vi "Datasheet Get Spara Result.vi"(5 "Frequency unit":string, 7 "Frequency":string, 8 "Run Information":T1, 9 "Type":T6, 10 "Format":T7=enum."SWR", 11 "Sxx":string) -> (3 "Table item":string)   [LabVIEW 2011]
uses:
  www/tests/S Parameter/TypeDefs/SP Format.ctl
  Datasheet Table Sxx Type.ctl
  TDMS/TDMS Run.ctl
  TDMS/TDMS Channel (Sxx).ctl
  database/Fields/Field Record.ctl
  database/Fields/Field DataTypes.ctl
  database/Fields/Field NextItem.ctl
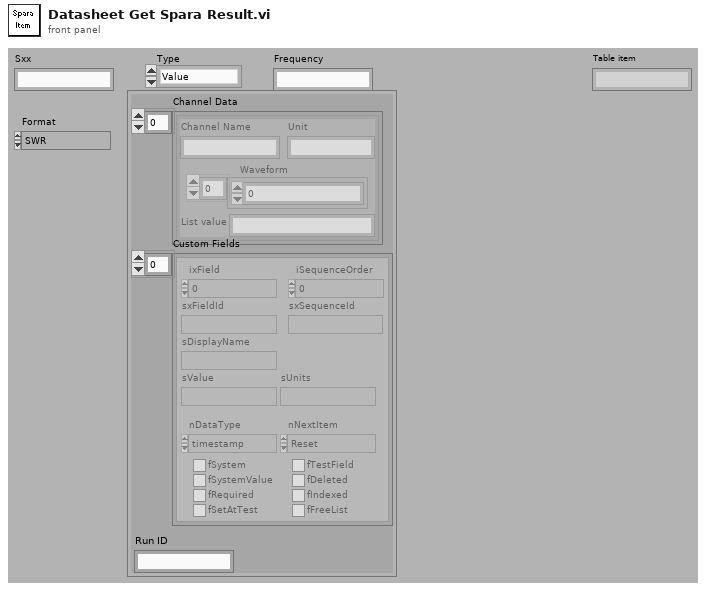
[diagram p1: front panel]
types:
  T1 = typedef "TDMS Run.ctl" = cluster{"Channel Data":T2[], "Custom Fields":T3[], "Run ID":string}
  T2 = typedef "TDMS Channel (Sxx).ctl" = cluster{"Channel Name":string, "Waveform":dbl[], "Unit":string, "List value":string}
  T3 = typedef "Field Record.ctl" = cluster{"ixField":i32, "iSequenceOrder":i32, "sxFieldId":string, "sxSequenceId":string, "sDisplayName":string, "sValue":string, "sUnits":string, "nDataType":T4, "nNextItem":T5, "fSystem":bool, "fSystemValue":bool, "fRequired":bool, "fSetAtTest":bool, "fTestField":bool, "fDeleted":bool, "fIndexed":bool, "fFreeList":bool}
  T4 = typedef "Field DataTypes.ctl" = enum32{"text", "numeric", "list", "timestamp", "boolean"}
  T5 = typedef "Field NextItem.ctl" = enum32{"Reset", "Retain", "Auto-Increment"}
  T6 = typedef "datasheet table Sxx type.ctl" = enum16{"Value", "Maximum", "Minimum", "Max Freq", "maxlimit", "minlimit", "Min Freq", "maxfreqlimit", "minfreqlimit"}
  T7 = typedef "SP Format.ctl" = enum16{"Log Mag", "Lin Mag", "SWR", "Phase", "Expanded Phase", "Delay", "Insertion Loss", "Isolation", "Return Loss"}
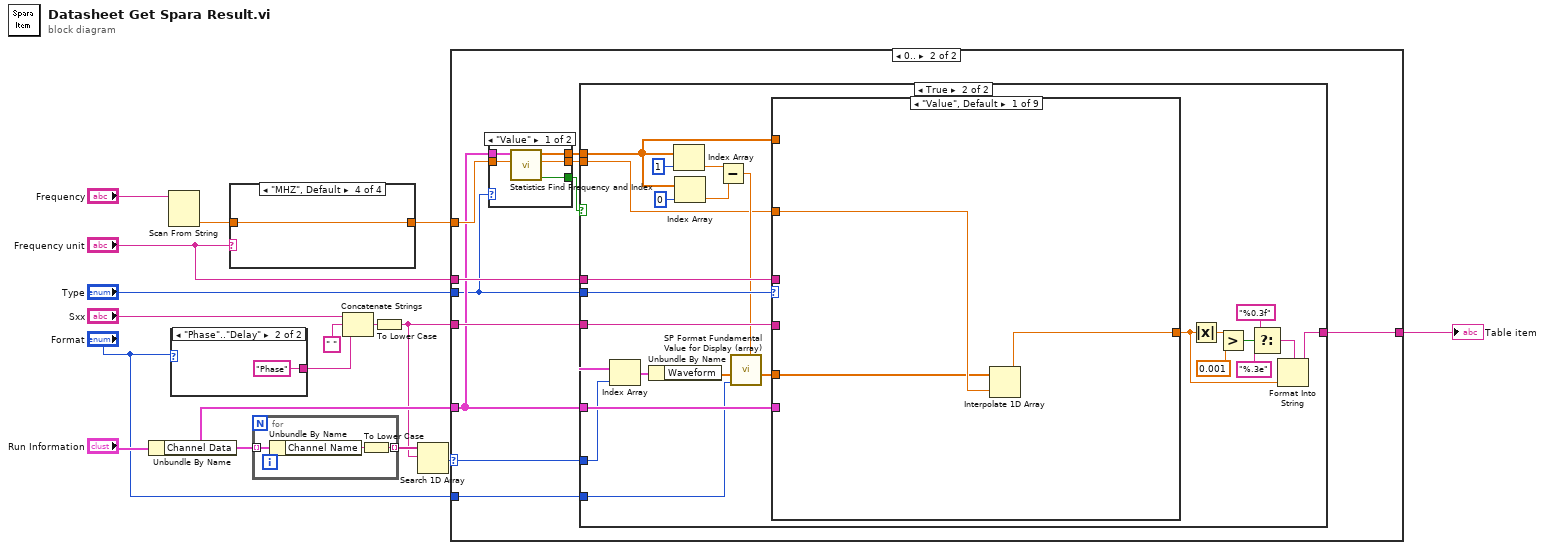
[diagram p0: block diagram]
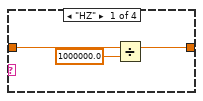
[diagram p2: hidden frame]
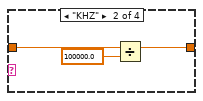
[diagram p3: hidden frame]
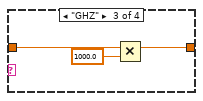
[diagram p4: hidden frame]
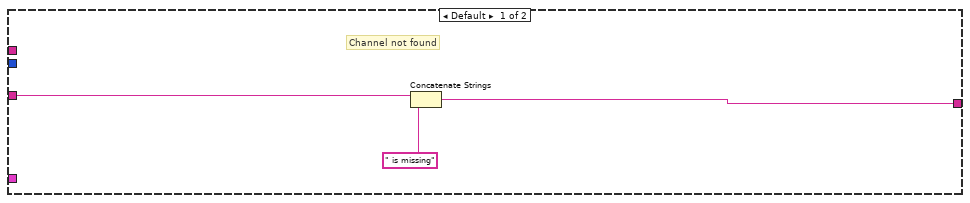
[diagram p5: hidden frame]
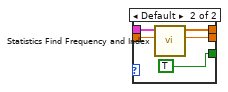
[diagram p6: hidden frame]
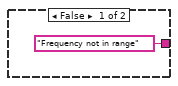
[diagram p7: hidden frame]
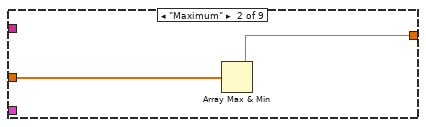
[diagram p8: hidden frame]
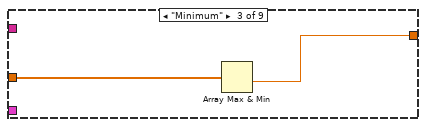
[diagram p9: hidden frame]
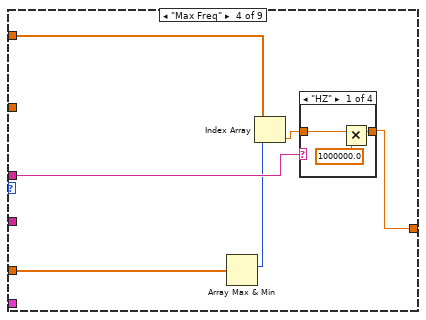
[diagram p10: hidden frame]
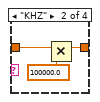
[diagram p11: hidden frame]
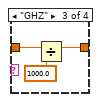
[diagram p12: hidden frame]
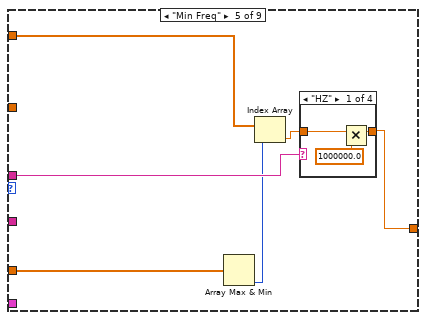
[diagram p14: hidden frame]
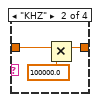
[diagram p15: hidden frame]
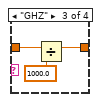
[diagram p16: hidden frame]
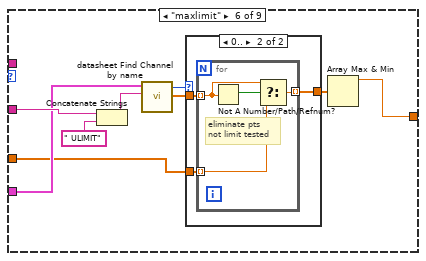
[diagram p18: hidden frame]
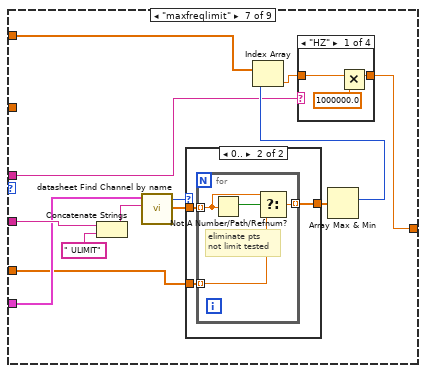
[diagram p20: hidden frame]
diagram:
  n1 = Unbundle By Name("Run Information") -> ("Channel Data"=w4:T2[])
  n2 = Scan From String(input string="Frequency") -> (output 1=w6:dbl)  [unwired: 3 in, 4 out]
  n3 = case shown="\"Phase\"..\"Delay\"" "Format" {
    tunnel: ["Mag" "Phase"] -> w16
    frame Default {
    }
    frame "Phase".."Delay" {
    }
  }
  n4 = case shown="\"MHZ\", Default" "Frequency unit" {
    tunnel: w6 -> [w21 w24 w27 w28]
    tunnel: [w20 w23 w26 w28] -> w5
    frame "HZ" {
      n5 = Divide(x=w21, y=1000000.0) -> (x/y=w20:dbl)
    }
    frame "KHZ" {
      n6 = Divide(x=w24, y=100000.0) -> (x/y=w23:dbl)
    }
    frame "GHZ" {
      n7 = Multiply(x=w27, y=1000.0) -> (x*y=w26:dbl)
    }
    frame "MHZ", Default {
    }
  }
  n8 = for {
    tunnel: w4 -> [w31] mode=indexing
    tunnel: [w29] -> w13 mode=indexing
    n9 = Unbundle By Name(w31) -> ("Channel Name"=w30:string)
    n10 = To Lower Case(string=w30) -> (all lower case string=w29:string)
  }
  n11 = Concatenate Strings("Sxx", " ", w16) -> (w10:string)
  n12 = To Lower Case(string=w10) -> (all lower case string=w3:string)
  n13 = Search 1D Array(1D array=w13, element=w3) -> (index of element=w11:i32)  [unwired: 1 out]
  n14 = case shown="0.." w11 {
    selector: w11 -> [_ w40]
    tunnel: w3 -> [w34 w43]
    tunnel: [w33 w44] -> w9
    tunnel: "Type" -> [_ w35]
    tunnel: w5 -> [_ w42]
    tunnel: w4 -> [_ w41]
    tunnel: "Format" -> [_ w38]
    tunnel: "Frequency unit" -> [_ w45]
    frame Default {
      # "Channel not found"
      n15 = Concatenate Strings(w34, " is missing") -> (w33:string)
    }
    frame 0.. {
      n16 = case shown="\"Value\"" w35 {
        tunnel: w42 -> [w50 w55]
        tunnel: w41 -> [w49 w54]
        tunnel: [w48 w53] -> w39
        tunnel: [w47 w52] -> w37
        tunnel: [w46 TRUE ("In Range?")] -> w36
        frame "Value" {
          n17 = call "Statistics Find Frequency and Index.vi"("MHz"=w50, "Channel Data"=w49) -> ("In Range?"=w46:bool, "Frequency Index"=w48:dbl, "Frequency Array"=w47:dbl[])  [unwired: 7 out]
        }
        frame Default {
          n18 = call "Statistics Find Frequency and Index.vi"("MHz"=w55, "Channel Data"=w54) -> ("Frequency Index"=w53:dbl, "Frequency Array"=w52:dbl[])  [unwired: 8 out]
        }
      }
      n19 = case shown="True" w36 {
        tunnel: w45 -> [_ w80]
        tunnel: ["Frequency not in range" w74] -> w44
        tunnel: w35 -> [_ w72]
        tunnel: w43 -> [_ w71]
        tunnel: w41 -> [_ w64]
        tunnel: w40 -> [_ w63]
        tunnel: w39 -> [_ w61]
        tunnel: w38 -> [_ w60]
        tunnel: w37 -> [_ w58]
        frame False {
        }
        frame True {
          n20 = Index Array(array=w64, index=w63) -> (element=w66:T2)
          n21 = Unbundle By Name(w66) -> ("Waveform"=w65:dbl[])
          n22 = Index Array(array=w58, index=1) -> (element=w68:dbl)
          n23 = Index Array(array=w58, index=0) -> (element=w67:dbl)
          n24 = Subtract(x=w68, y=w67) -> (x-y=w62:dbl)
          n25 = call "SP Format Fundamental Value for Display (array).vi"("dF, MHz"=w62, "Display Format"=w60, "Fundamental Values"=w65) -> ("Formatted Values"=w59:dbl[])  [unwired: 1 in, 7 out]
          n26 = case shown="\"Value\", Default" w72 {
            tunnel: w80 -> [_ _ _ w93 w109 _ w139 _ w187]
            tunnel: w64 -> [_ _ _ _ _ w124 w146 w173 w194]
            tunnel: [w83 w85 w87 w92 w108 w125 w141 w169 w188] -> w73
            tunnel: w71 -> [_ _ _ _ _ w127 w148 w175 w196]
            tunnel: w61 -> [w82 _ _ _ _ _ _ _ _]
            tunnel: w59 -> [w81 w84 w86 w88 w104 w120 w137 w168 w185]
            tunnel: w58 -> [_ _ _ w89 w105 _ w138 _ w186]
            frame "Value", Default {
              n27 = Interpolate 1D Array(1:w82, 2:w81) -> (0:w83:dbl)
            }
            frame "Maximum" {
              n28 = Array Max & Min(array=w84) -> (max value=w85:dbl)  [unwired: 3 out]
            }
            frame "Minimum" {
              n29 = Array Max & Min(array=w86) -> (min value=w87:dbl)  [unwired: 3 out]
            }
            frame "Max Freq" {
              n30 = Array Max & Min(array=w88) -> (max index (indices)=w91:i32)  [unwired: 3 out]
              n31 = Index Array(array=w89, index=w91) -> (element=w90:dbl)
              n32 = case shown="\"HZ\"" w93 {
                tunnel: w90 -> [w96 w99 w102 w103]
                tunnel: [w95 w98 w101 w103] -> w92
                frame "HZ" {
                  n33 = Multiply(x=w96, y=1000000.0) -> (x*y=w95:dbl)
                }
                frame "KHZ" {
                  n34 = Multiply(x=w99, y=100000.0) -> (x*y=w98:dbl)
                }
                frame "GHZ" {
                  n35 = Divide(x=w102, y=1000.0) -> (x/y=w101:dbl)
                }
                frame "MHZ", Default {
                }
              }
            }
            frame "Min Freq" {
              n36 = Array Max & Min(array=w104) -> (min index (indices)=w106:i32)  [unwired: 3 out]
              n37 = Index Array(array=w105, index=w106) -> (element=w107:dbl)
              n38 = case shown="\"HZ\"" w109 {
                tunnel: w107 -> [w112 w115 w118 w119]
                tunnel: [w111 w114 w117 w119] -> w108
                frame "HZ" {
                  n39 = Multiply(x=w112, y=1000000.0) -> (x*y=w111:dbl)
                }
                frame "KHZ" {
                  n40 = Multiply(x=w115, y=100000.0) -> (x*y=w114:dbl)
                }
                frame "GHZ" {
                  n41 = Divide(x=w118, y=1000.0) -> (x/y=w117:dbl)
                }
                frame "MHZ", Default {
                }
              }
            }
            frame "maxlimit" {
              n42 = Concatenate Strings(w127, " ULIMIT") -> (w123:string)
              n43 = call "datasheet Find Channel by name.vi"("Channel Name"=w123, "Channel Data"=w124) -> ("Waveform"=w122:dbl[], "index of element"=w121:i32)  [unwired: 8 out]
              n44 = case shown="0.." w121 {
                tunnel: w120 -> [w129 w132]
                tunnel: [w129 w131] -> w126
                tunnel: w122 -> [_ w130]
                frame -1, Default {
                  # "did not find\nlimit"
                }
                frame 0.. {
                  n45 = for {
                    tunnel: w130 -> [w135] mode=indexing
                    tunnel: w132 -> [w134] mode=indexing
                    tunnel: [w133] -> w131 mode=indexing
                    # "eliminate pts \nnot limit tested"
                    n46 = Not A Number/Path/Refnum?(number/path/refnum=w135) -> (NaN/Path/Refnum?=w136:bool)
                    n47 = Select(t=w135, s=w136, f=w134) -> (s? t:f=w133:dbl)
                  }
                }
              }
              n48 = Array Max & Min(array=w126) -> (max value=w125:dbl)  [unwired: 3 out]
            }
            frame "maxfreqlimit" {
              n49 = Concatenate Strings(w148, " ULIMIT") -> (w145:string)
              n50 = call "datasheet Find Channel by name.vi"("Channel Name"=w145, "Channel Data"=w146) -> ("Waveform"=w144:dbl[], "index of element"=w143:i32)  [unwired: 8 out]
              n51 = case shown="0.." w143 {
                tunnel: w137 -> [w160 w163]
                tunnel: [w160 w162] -> w147
                tunnel: w144 -> [_ w161]
                frame -1, Default {
                  # "did not find\nlimit"
                }
                frame 0.. {
                  n52 = for {
                    tunnel: w161 -> [w166] mode=indexing
                    tunnel: w163 -> [w165] mode=indexing
                    tunnel: [w164] -> w162 mode=indexing
                    # "eliminate pts \nnot limit tested"
                    n53 = Not A Number/Path/Refnum?(number/path/refnum=w166) -> (NaN/Path/Refnum?=w167:bool)
                    n54 = Select(t=w166, s=w167, f=w165) -> (s? t:f=w164:dbl)
                  }
                }
              }
              n55 = Array Max & Min(array=w147) -> (max index (indices)=w140:i32)  [unwired: 3 out]
              n56 = Index Array(array=w138, index=w140) -> (element=w142:dbl)
              n57 = case shown="\"HZ\"" w139 {
                tunnel: w142 -> [w152 w155 w158 w159]
                tunnel: [w151 w154 w157 w159] -> w141
                frame "HZ" {
                  n58 = Multiply(x=w152, y=1000000.0) -> (x*y=w151:dbl)
                }
                frame "KHZ" {
                  n59 = Multiply(x=w155, y=100000.0) -> (x*y=w154:dbl)
                }
                frame "GHZ" {
                  n60 = Divide(x=w158, y=1000.0) -> (x/y=w157:dbl)
                }
                frame "MHZ", Default {
                }
              }
            }
            frame "minlimit" {
              n61 = Concatenate Strings(w175, " LLIMIT") -> (w172:string)
              n62 = call "datasheet Find Channel by name.vi"("Channel Name"=w172, "Channel Data"=w173) -> ("Waveform"=w171:dbl[], "index of element"=w170:i32)  [unwired: 8 out]
              n63 = case shown="0.." w170 {
                tunnel: w168 -> [w177 w180]
                tunnel: [w177 w179] -> w174
                tunnel: w171 -> [_ w178]
                frame -1, Default {
                  # "did not find\nlimit"
                }
                frame 0.. {
                  n64 = for {
                    tunnel: w178 -> [w183] mode=indexing
                    tunnel: w180 -> [w182] mode=indexing
                    tunnel: [w181] -> w179 mode=indexing
                    # "eliminate pts \nnot limit tested"
                    n65 = Not A Number/Path/Refnum?(number/path/refnum=w183) -> (NaN/Path/Refnum?=w184:bool)
                    n66 = Select(t=w183, s=w184, f=w182) -> (s? t:f=w181:dbl)
                  }
                }
              }
              n67 = Array Max & Min(array=w174) -> (min value=w169:dbl)  [unwired: 3 out]
            }
            frame "minfreqlimit" {
              n68 = Concatenate Strings(w196, " LLIMIT") -> (w193:string)
              n69 = call "datasheet Find Channel by name.vi"("Channel Name"=w193, "Channel Data"=w194) -> ("Waveform"=w192:dbl[], "index of element"=w191:i32)  [unwired: 8 out]
              n70 = case shown="0.." w191 {
                tunnel: w185 -> [w208 w211]
                tunnel: [w208 w210] -> w195
                tunnel: w192 -> [_ w209]
                frame -1, Default {
                  # "did not find\nlimit"
                }
                frame 0.. {
                  n71 = for {
                    tunnel: w209 -> [w214] mode=indexing
                    tunnel: w211 -> [w213] mode=indexing
                    tunnel: [w212] -> w210 mode=indexing
                    # "eliminate pts \nnot limit tested"
                    n72 = Not A Number/Path/Refnum?(number/path/refnum=w214) -> (NaN/Path/Refnum?=w215:bool)
                    n73 = Select(t=w214, s=w215, f=w213) -> (s? t:f=w212:dbl)
                  }
                }
              }
              n74 = Array Max & Min(array=w195) -> (min index (indices)=w189:i32)  [unwired: 3 out]
              n75 = Index Array(array=w186, index=w189) -> (element=w190:dbl)
              n76 = case shown="\"HZ\"" w187 {
                tunnel: w190 -> [w200 w203 w206 w207]
                tunnel: [w199 w202 w205 w207] -> w188
                frame "HZ" {
                  n77 = Multiply(x=w200, y=1000000.0) -> (x*y=w199:dbl)
                }
                frame "KHZ" {
                  n78 = Multiply(x=w203, y=100000.0) -> (x*y=w202:dbl)
                }
                frame "GHZ" {
                  n79 = Divide(x=w206, y=1000.0) -> (x/y=w205:dbl)
                }
                frame "MHZ", Default {
                }
              }
            }
          }
          n80 = Absolute Value(x=w73) -> (abs(x)=w57:dbl)
          n81 = Greater?(x=w57, y=0.001) -> (0:w78:bool)
          n82 = Select(t="%0.3f" ("format string"), s=w78, f="%.3e" ("format string")) -> (s? t:f=w76:string)
          n83 = Format Into String(format string=w76, w73) -> (resulting string=w74:string)  [unwired: 2 in, 1 out]
        }
      }
    }
  }
  "Table item" <- w9
